vi "resource_array_size_greater_than_zero.vi"(10 "Resources in":refnum<k20>[](array[refnum])) -> (2 "array size >0?":bool)   [LabVIEW 2015]
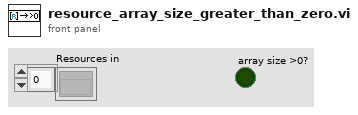
[diagram p1: front panel]
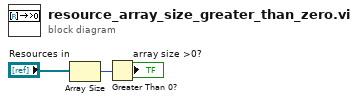
[diagram p0: block diagram]
diagram:
  n1 = Array Size(array="Resources in") -> (size(s)=w2:i32)
  n2 = Greater Than 0?(x=w2) -> (x > 0?=→"array size >0?":bool)
